vi "Clear Digital Audio Task.vi"(8 "error in (no error)":errorcluster, 10 "master clock task":T1, 11 "data task":T1) -> (0 "error out":errorcluster)   [LabVIEW 2021, in "DigitalAudioGenerationProcess.lvlib"]
uses:
  <vilib>/PDM Acquisition Toolkit/host/Classes/Tasks/PCM Output/Controls/PCM Output Task DVR.ctl
  <vilib>/PDM Acquisition Toolkit/host/Classes/Tasks/PCM Output/PCM Output Task.lvclass
  DigitalAudioGenerationProcess.lvlib
  <vilib>/PDM Acquisition Toolkit/host/API/PDM Acquisition Toolkit.lvlib
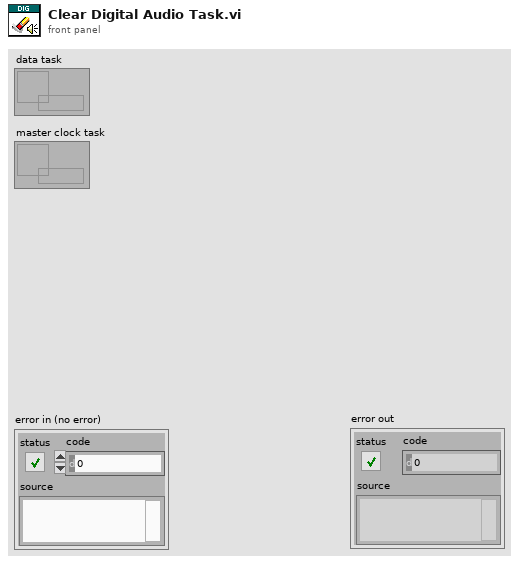
[diagram p1: front panel]
types:
  T1 = typedef "PDM Acquisition Class Library.lvlib/PCM Output Task.lvclass/PCM Output Task DVR.ctl" = refnum<data-value>
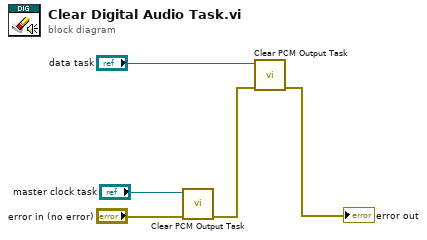
[diagram p0: block diagram]
diagram:
  n1 = call <vilib>:"Clear PCM Output Task.vi"("error in"="error in (no error)", "PCM output task in"="master clock task") -> ("error out"=w3:errorcluster)  [unwired: 9 in]
  n2 = call <vilib>:"Clear PCM Output Task.vi"("error in"=w3, "PCM output task in"="data task") -> ("error out"=→"error out":errorcluster)  [unwired: 9 in]
